vi "Write Error.vi"(1 "Message To Write":string, 2 "Error Code":i32) -> (0 "error out":errorcluster)   [LabVIEW 2017]
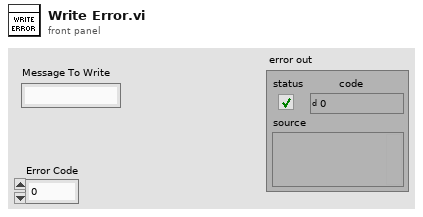
[diagram p1: front panel]
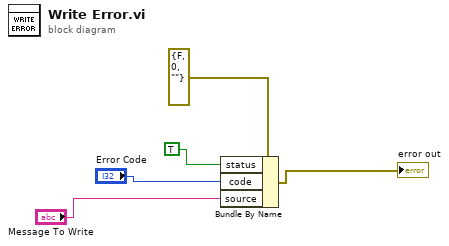
[diagram p0: block diagram]
diagram:
  n1 = Bundle By Name(cluster=errorcluster {"status"=FALSE, "code"=0, "source"=""} ("error out"), "status"=TRUE, "code"="Error Code", "source"="Message To Write") -> (→"error out":errorcluster)
